vi "SRTS_Header.vi"(8 "error in":errorcluster, 10 "date":string, 11 "XLS in":refnum<class "XLS.lvclass">=refnum) -> (0 "error out":errorcluster, 3 "XLS out":refnum<class "XLS.lvclass">)   [LabVIEW 2017, in "Report_lib.lvlib" / "XLS.lvclass"]
doc: "This method performs and fullfill\ncommon Header for XLS report"
uses:
  XLS.lvclass
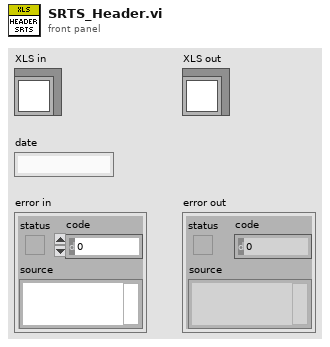
[diagram p1: front panel]
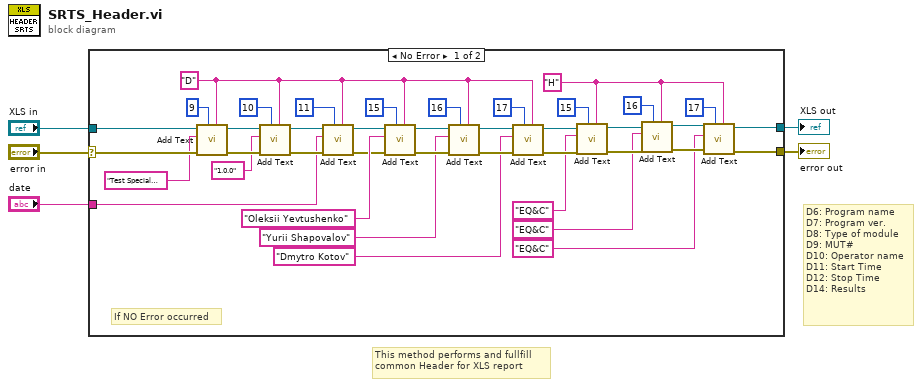
[diagram p0: block diagram]
diagram:
  # "This method performs and fullfill\ncommon Header for XLS report"
  # "D6: Program name\nD7: Program ver.\nD8: Type of module\nD9: MUT#\nD10: Operator name\nD11: Start Time\nD12: Stop Time\nD14: Results"
  n1 = case shown="No Error" "error in" {
    selector: "error in" -> [w45 w47]
    tunnel: [w27 w47] -> w4
    tunnel: [w28 w46] -> w2
    tunnel: "XLS in" -> [w44 w46]
    tunnel: "date" -> [w6 _]
    frame No Error {
      w19 = "H" ("Adr")
      w7 = "D" ("Adr")
      # "If NO Error occurred"
      n2 = call "Add Text.vi"("Adr"=w7, "Index"=9, "error in"=w45, "text"="Test Special Program", "XLS in"=w44) -> ("error out"=w41:errorcluster, "XLS out"=w42:refnum<class "XLS.lvclass">)  [unwired: 5 in]
      n3 = call "Add Text.vi"("Adr"=w7, "Index"=10, "error in"=w41, "text"="1.0.0", "XLS in"=w42) -> ("error out"=w12:errorcluster, "XLS out"=w9:refnum<class "XLS.lvclass">)  [unwired: 5 in]
      n4 = call "Add Text.vi"("Adr"=w7, "Index"=11, "error in"=w12, "text"=w6, "XLS in"=w9) -> ("error out"=w11:errorcluster, "XLS out"=w10:refnum<class "XLS.lvclass">)  [unwired: 5 in]
      n5 = call "Add Text.vi"("Adr"=w7, "Index"=15, "error in"=w11, "text"="Oleksii Yevtushenko", "XLS in"=w10) -> ("error out"=w36:errorcluster, "XLS out"=w37:refnum<class "XLS.lvclass">)  [unwired: 5 in]
      n6 = call "Add Text.vi"("Adr"=w7, "Index"=16, "error in"=w36, "text"="Yurii Shapovalov", "XLS in"=w37) -> ("error out"=w33:errorcluster, "XLS out"=w34:refnum<class "XLS.lvclass">)  [unwired: 5 in]
      n7 = call "Add Text.vi"("Adr"=w7, "Index"=17, "error in"=w33, "text"="Dmytro Kotov", "XLS in"=w34) -> ("error out"=w31:errorcluster, "XLS out"=w30:refnum<class "XLS.lvclass">)  [unwired: 5 in]
      n8 = call "Add Text.vi"("Adr"=w19, "Index"=15, "error in"=w31, "text"="EQ&C", "XLS in"=w30) -> ("error out"=w22:errorcluster, "XLS out"=w23:refnum<class "XLS.lvclass">)  [unwired: 5 in]
      n9 = call "Add Text.vi"("Adr"=w19, "Index"=16, "error in"=w22, "text"="EQ&C", "XLS in"=w23) -> ("error out"=w20:errorcluster, "XLS out"=w21:refnum<class "XLS.lvclass">)  [unwired: 5 in]
      n10 = call "Add Text.vi"("Adr"=w19, "Index"=17, "error in"=w20, "text"="EQ&C", "XLS in"=w21) -> ("error out"=w27:errorcluster, "XLS out"=w28:refnum<class "XLS.lvclass">)  [unwired: 5 in]
    }
    frame Error {
    }
  }
  "error out" <- w4
  "XLS out" <- w2
